vi "Tetra_BOUNCE_Payload.vi"(8 "error in":errorcluster, 10 "Input Constants":string[](array[string]), 11 "Parameters":string[](array[string])=["room", "18.75", "1", "0", "1", "15.5", "31.5"]) -> (0 "error out":errorcluster={"status"=FALSE, "code"=1073676294, "source"="VISA Read in Tetra Loop Serial.vi:4650001->Tetra_Read Imon.vi->Tetra_TX_Payload.vi"}, 2 "Payload Results":string[](array[string])=["0.000", "0.000", "0.000", "0.000", "0.000", "0.000", "0.000", "0.000", "-32.000", "1.000", "18.390", "0.998", "1.810", "3.312", "0.996", "1.198", "5.011", "3.316", "2.513", "2.513", "3.600", "5.496", "2.776", "2.768", "2.280", "1.360", "0.187", "0.089", "0.321", "0.340", "1.483", "0.530", "0.827", "7.000", "P0003", "trace file path"])   [LabVIEW 2018]
uses:
  778a857b-ea1c-4c41-85f0-8bde546241f8.vi
  e7e3a4d5-9ed6-4285-8f90-f7af1205463a.vi
  Initialize References/Station References Global.vi
  Initialize References/Sequence Globals.vi
  Tetra_Globals.vi
  Infrastructure/Test Parameter Globals_1.0.0.vi
  Infrastructure/Test Result File Name Global.vi
panel:
  in  "Controls":T1={"ReadADC"=TRUE, "StartTest"=TRUE, "ResetRFSM"=TRUE, "FtServer"=TRUE, "CalVCO(t)"=TRUE, "Ping(t)"=TRUE, "CmdWindowHide(T)"=FALSE, "OpenNewFt(T)"=TRUE, "UseCmdFile(T)"=FALSE, "#of Retries"=5}
  out "message":string="Scan Failed! Try to run vco cal, then press OK\nScan Failed! In Field Test ; Try to Terminate Scan, Then Prep for new scan"
  out "Pass?(T)":bool
  out "Current Iteration":i32=1
  out "PASS/FAIL":string
  out "DataToResultFile":string[][](array[string])
  out "no_fault":bool
  out "FH_NOT(T)":bool
  in  "ess_error":errorcluster
  out "STOP(T)":bool
  in  "Tab Control":enum32{"Page 1", "Page 2", "Page 3", "Page 4"}(tab)
  out "#OFAVGs":i32
  out "Temp Soak(min)":dbl
  in  "Standalone(T)":bool
  out "V_SUPPLY(t)":bool
  out "TEMP(t)":bool
  out "GET_TRACE":bool
  out "TEMP":dbl
  out "V_SUPPLY":dbl=18.75
  in  "CheckDataRetry(t)":bool
  out "ps_meas(i)(w)":dbl[](array[numeric])
  out "Ampl_Graph":dbl[][](graph)
  out "Freq_Graph":dbl[](graph)
  out "comport":refnum<visa-resource-name>
  out "CalFileA":path
  out "relative seconds":dbl=73640.4138221 format="%_19f"
  out "iq_file_str":string
  out "TraceFilePath":path
  out "Run_Clk_Test(t)":bool
  out "ClkTestPASS?(t)":bool
  out "PyScript(path)":path=path "C:/RageATE/Automated Tests/Tetra WAM/Utilities/VerifySiTime.py"
  out "WamGood(path)":path=path "C:/RageATE/Automated Tests/Tetra WAM/Utilities/ext_wamGood.txt"
  out "CLK_P/F(str)":string
  out "GuiPath":path
  out "FtPath":path
  # "Globals (last value change)"
  # "Vmon & Imon"
  # "Temp Sensors"
types:
  T1 = cluster{"ReadADC":bool, "StartTest":bool, "ResetRFSM":bool, "FtServer":bool, "CalVCO(t)":bool, "Ping(t)":bool, "CmdWindowHide(T)":bool, "OpenNewFt(T)":bool, "UseCmdFile(T)":bool, "#of Retries":i32}
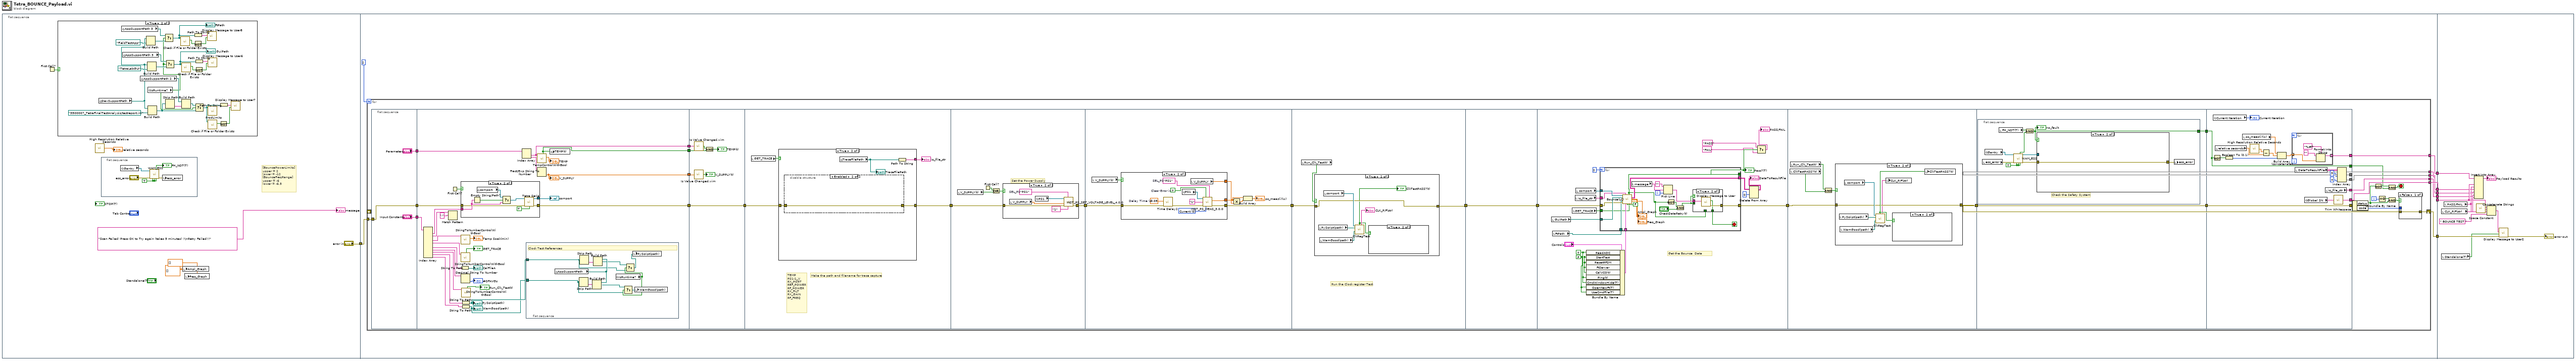
[diagram p0: block diagram]
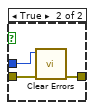
[diagram p3: hidden frame]
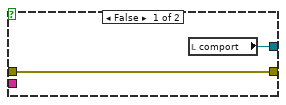
[diagram p4: hidden frame]
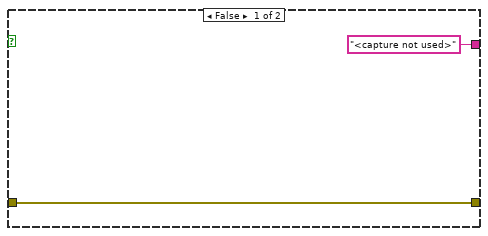
[diagram p5: hidden frame]
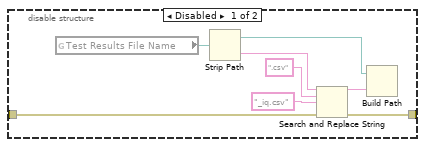
[diagram p6: hidden frame]
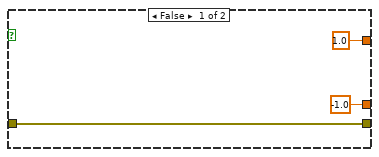
[diagram p8: hidden frame]
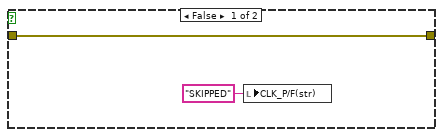
[diagram p9: hidden frame]
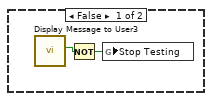
[diagram p10: hidden frame]
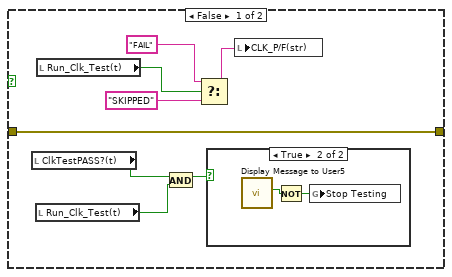
[diagram p12: hidden frame]
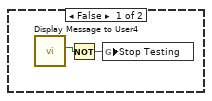
[diagram p14: hidden frame]
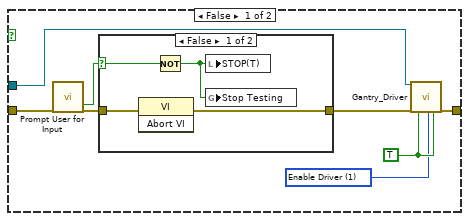
[diagram p15: hidden frame]
diagram:
  n1 = flat-sequence {
    tunnel: ["error in"] -> w5
    tunnel: [w51] -> w7
    tunnel: [w50] -> w6
    tunnel: w5 -> [w49]
    tunnel: [w47] -> w4
    tunnel: [w46] -> w3
    tunnel: [w45] -> w2
    tunnel: [w44] -> w1
    tunnel: w1 -> [w332]
    tunnel: w2 -> [w333]
    tunnel: w3 -> [w334]
    tunnel: w4 -> [w336]
    tunnel: w6 -> [w335]
    tunnel: w7 -> [w337]
    frame #0 {
      # "[BouncePowerLimits]\nupper = 2\nlower = -12\n[BounceFreqRange]\nupper = -6\nlower = -6.5"
      n2 = First Call?() -> (First Call?: T/F=w11:bool)
      n3 = case shown="True" w11 {
        frame False {
        }
        frame True {
          n4 = global read "Sequence Globals.vi" "DevSupportPath"() -> (w15:path)
          n5 = global read "Sequence Globals.vi" "AppSupportPath 3"() -> (w16:path)
          n6 = global read "Sequence Globals.vi" "AppSupportPath 3"() -> (w35:path)
          n7 = global read "Sequence Globals.vi" "AppSupportPath 2"() -> (w37:path)
          n8 = Build Path(base path=w15, name or relative path=path "FieldTestApp" ("*.ini file")) -> (appended path=w17:path)
          n9 = Build Path(base path=w15, name or relative path=path "TetraLabGUI" ("*.ini file")) -> (appended path=w32:path)
          n10 = global read "Sequence Globals.vi" "IsRuntime?"() -> (w14:bool)
          n11 = Build Path(base path=w15, name or relative path=path "3500007_TetraFinalTestAnalysis/testreport.ini" ("*.ini file")) -> (appended path=w34:path)
          n12 = Select(t=w16, s=w14, f=w17) -> (s? t:f=w19:path)
          "FtPath" <- w19
          n13 = Select(t=w35, s=w14, f=w32) -> (s? t:f=w30:path)
          "GuiPath" <- w30
          n14 = Strip Path(path=w34) -> (name=w38:string)  [unwired: 1 out]
          n15 = call <vilib>:"Check if File or Folder Exists.vi"("path"=w19) -> ("file or folder exists?"=w21:bool)  [unwired: 8 in, 2 out]
          n16 = call <vilib>:"Check if File or Folder Exists.vi"("path"=w30) -> ("file or folder exists?"=w24:bool)  [unwired: 8 in, 2 out]
          n17 = Build Path(base path=w37, name or relative path=w38) -> (appended path=w36:path)
          n18 = Path To String(path=w19) -> (string=w20:string)
          n19 = Not(x=w21) -> (.not. x?=w22:bool)
          n20 = Path To String(path=w30) -> (string=w29:string)
          n21 = Not(x=w24) -> (.not. x?=w23:bool)
          n22 = Select(t=w36, s=w14, f=w34) -> (s? t:f=w27:path)
          n23 = call "Display Message to User8"("Enable"=w22, "Message"=w20) -> ()  [unwired: 8 in, 2 out]
          n24 = call "Display Message to User6"("Enable"=w23, "Message"=w29) -> ()  [unwired: 8 in, 2 out]
          n25 = call "ProdLimits.vi"("*.ini file"=w27) -> ()  [unwired: 9 in, 2 out]
          n26 = call <vilib>:"Check if File or Folder Exists.vi"("path"=w27) -> ("file or folder exists?"=w26:bool)  [unwired: 8 in, 2 out]
          n27 = Path To String(path=w27) -> (string=w28:string)
          n28 = Not(x=w26) -> (.not. x?=w25:bool)
          n29 = call "Display Message to User7"("Enable"=w25, "Message"=w28) -> ()  [unwired: 8 in, 2 out]
        }
      }
      n30 = call <vilib>:"High Resolution Relative Seconds.vi"() -> ("relative seconds"=→"relative seconds":dbl)
      n31 = flat-sequence {
        frame #0 {
          w41 = TRUE ("Test Running (T)")
          n32 = global read "Station References Global.vi" "Gantry"() -> (w42:refnum<visa-resource-name>)
          n33 = call "WAM_ESS.vi"("VISA resource name"=w42, "error in (no error)"="ess_error", "Open Serial"=w41, "Test Running (T)"=w41, "Close Serial"=w41) -> ("FH_NOT(T)"=→"FH_NOT(T)":bool, "error out"=w39:errorcluster)  [unwired: 7 in, 2 out]
          n34 = local write "ess_error"(w39) -> ()
        }
      }
      n35 = local write "Ampl_Graph"(dbl[][] [] ("Ampl_Graph")) -> ()
      n36 = local write "Freq_Graph"(dbl[] [] ("Freq_Graph")) -> ()
      "message" <- "Scan Failed! Press OK to Try again (takes 5 minutes) !!\nRetry Failed!!!" ("multi-line string")
    }
    frame #1 {
      n37 = for {
        N: 2 -> [_]
        tunnel: [w75] -> w51
        tunnel: [w74] -> w50
        tunnel: w49 -> [w73]
        shift-right: [w68] -> w47
        shift-left: _ -> [_]
        tunnel: [w61] -> w46
        tunnel: [w60] -> w45
        tunnel: [w59] -> w44
        i -> [w65]
        stop <- w71 stop-if-true
        n38 = flat-sequence {
          tunnel: [w89] -> w84
          tunnel: ["Parameters"] -> w83
          tunnel: ["Input Constants"] -> w82
          tunnel: w73 -> [w89]
          tunnel: w84 -> [w100]
          tunnel: [w99] -> w81
          tunnel: w83 -> [w114]
          tunnel: w82 -> [w113]
          tunnel: [w112] -> w80
          tunnel: [w109] -> w79
          tunnel: [w104] -> w78
          tunnel: [w146] -> w77
          tunnel: w78 -> [w140]
          tunnel: w79 -> [w142]
          tunnel: w80 -> [w144]
          tunnel: w81 -> [w146]
          tunnel: [w149] -> w72
          tunnel: w77 -> [w148]
          tunnel: [w170] -> w76
          tunnel: w72 -> [w168]
          tunnel: [w184] -> w55
          tunnel: w76 -> [w183]
          tunnel: w55 -> [w201]
          tunnel: [w200] -> w54
          tunnel: w54 -> [w212]
          tunnel: [w212] -> w58
          tunnel: [w229] -> w53
          tunnel: w58 -> [w231]
          tunnel: w53 -> [w260]
          tunnel: [w261] -> w52
          tunnel: w52 -> [w280]
          tunnel: [w281] -> w62
          tunnel: [w280] -> w56
          tunnel: [w315] -> w67
          tunnel: [w320] -> w75
          tunnel: [w317] -> w74
          tunnel: w62 -> [w305]
          tunnel: [w310] -> w61
          tunnel: [w308] -> w60
          tunnel: [w307] -> w59
          tunnel: [w305] -> w57
          tunnel: w56 -> [w315]
          frame #0 {
          }
          frame #1 {
            n39 = Index Array(array=w113) -> (element #1=w102:string, element #2=w105:string, element #4=w119:string, element #5=w98:string, element #7=w116:string, element #8=w111:string, element #9=w97:string, element #10=w95:string, element #11=w94:string)  [unwired: 11 in, 2 out]
            n40 = Match Pattern(string=w105, regular expression=";") -> ()  [unwired: 1 in, 4 out]
            n41 = First Call?() -> (First Call?: T/F=w101:bool)
            n42 = String To Path(string=w116) -> (path=→"CalFileA":path)
            n43 = case shown="True" w101 {
              tunnel: [w131 w135] -> w103
              tunnel: w102 -> [_ w137]
              tunnel: w100 -> [w130 w134]
              tunnel: [w130 w133] -> w99
              frame False {
                n44 = local read "comport"() -> (w131:refnum<visa-resource-name>)
              }
              frame True {
                n45 = Empty String/Path?(string/path=w137) -> (empty?=w139:bool)
                n46 = global read "Tetra_Globals.vi" "comport"() -> (w138:refnum<visa-resource-name>)
                n47 = Select(t=w138, s=w139, f=w137) -> (s? t:f=w136:refnum<visa-resource-name>)
                n48 = call "Tetra Serial.vi"("COMPORT"=w136, "error in (no error)"=w134, "Open Ser(t)"=TRUE) -> ("comport"=w135:refnum<visa-resource-name>, "error out"=w133:errorcluster)  [unwired: 8 in, 3 out]
              }
            }
            "comport" <- w103
            n49 = call "StringToNumberControlWithBool.vi"("String In"=w119) -> ("Number Out"=→"Temp Soak(min)":dbl)  [unwired: 7 in, 1 out]
            n50 = call "StringToNumberControlWithBool.vi"("String In"=w98) -> ("NOT = 0"=→"GET_TRACE":bool)  [unwired: 7 in, 1 out]
            n51 = Decimal String To Number(string=w111) -> (number=→"#OFAVGs":i32)  [unwired: 2 in, 1 out]
            n52 = String To Path(string=w95) -> (path=w93:path)
            "PyScript(path)" <- w93
            n53 = String To Path(string=w94) -> (path=w92:path)
            "WamGood(path)" <- w92
            n54 = call "StringToNumberControlWithBool.vi"("String In"=w97) -> ("NOT = 0"=→"Run_Clk_Test(t)":bool)  [unwired: 7 in, 1 out]
            n55 = Index Array(array=w114) -> (element #1=w109:string, element #2=w118:string)  [unwired: 2 in]
            n56 = flat-sequence {
              tunnel: w93 -> [w121]
              tunnel: w92 -> [w120]
              frame #0 {
                # "Clock Test References"
                n57 = global read "Sequence Globals.vi" "AppSupportPath"() -> (w127:path)
                n58 = Strip Path(path=w120) -> (name=w128:string)  [unwired: 1 out]
                n59 = Strip Path(path=w121) -> (name=w129:string)  [unwired: 1 out]
                n60 = Build Path(base path=w127, name or relative path=w128) -> (appended path=w125:path)
                n61 = Build Path(base path=w127, name or relative path=w129) -> (appended path=w126:path)
                n62 = global read "Sequence Globals.vi" "IsRuntime?"() -> (w124:bool)
                n63 = Select(t=w125, s=w124, f=w120) -> (s? t:f=w122:path)
                n64 = Select(t=w126, s=w124, f=w121) -> (s? t:f=w123:path)
                n65 = local write "PyScript(path)"(w123) -> ()
                n66 = local write "WamGood(path)"(w122) -> ()
              }
            }
            n67 = call "TempControlWithBool.vi"("INPUT"=w109) -> ("out"=→"TEMP":dbl, "Valid(t)"=w104:bool)  [unwired: 6 in, 1 out]
            n68 = Fract/Exp String To Number(string=w118) -> (number=w112:dbl)  [unwired: 3 in, 1 out]
            "V_SUPPLY" <- w112
            n69 = global write "Tetra_Globals.vi" "TEMP(t)"(w104) -> ()
          }
          frame #2 {
            n70 = call "Is Value Changed.vim"("value"=w142) -> ("changed or first call?"=w143:bool)
            n71 = call "Is Value Changed.vim"("value"=w144) -> ("changed or first call?"=→"V_SUPPLY(t)":bool)
            n72 = And(x=w143, y=w140) -> (x .and. y?=→"TEMP(t)":bool)
          }
          frame #3 {
            # "TEMP\nPS1-1_V\nRX_PORT\nREF_POWER\nRF_POWER\nRX_FILT\nRX_GAIN\nRF_FREQ"
            # "Make the path and filename for trace capture"
            n73 = local read "GET_TRACE"() -> (w150:bool)
            n74 = case shown="True" w150 {
              tunnel: [w152 w155] -> w149
              tunnel: w148 -> [w152 w156]
              tunnel: ["<capture not used>" w154] -> w147
              frame False {
              }
              frame True {
                n75 = disable-structure shown="Enabled" {
                  disable-tunnel: w156 -> [w158 w165]
                  disable-tunnel: [w157 w165] -> w155
                  frame Disabled {
                    n76 = global read "Test Result File Name Global.vi" "Test Results File Name"() -> (w161:path)
                    n77 = Strip Path(path=w161) -> (stripped path=w162:path, name=w164:string)
                    n78 = Search and Replace String(input string=w164, search string=".csv", replace string="_iq.csv" ("name or relative path"), error in=w158) -> (result string=w163:string, error out=w157:errorcluster)  [unwired: 4 in, 2 out]
                    n79 = Build Path(base path=w162, name or relative path=w163) -> ()  [unwired: 1 out]
                  }
                  frame Enabled {
                  }
                }
                n80 = global read "Tetra_Globals.vi" "TraceFilePath"() -> (w153:path)
                "TraceFilePath" <- w153
                n81 = Path To String(path=w153) -> (string=w154:string)
              }
            }
            "iq_file_str" <- w147
          }
          frame #4 {
            # "Set the Power Supply"
            n82 = local read "V_SUPPLY(t)"() -> (w169:bool)
            n83 = First Call?() -> (First Call?: T/F=w167:bool)
            n84 = Or(x=w167, y=w169) -> (x .or. y?=w166:bool)
            n85 = case shown="True" w166 {
              tunnel: [w171 w173] -> w170
              tunnel: w168 -> [w171 w172]
              frame False {
              }
              frame True {
                w176 = "PS1"  # SEL_PS
                n86 = local read "V_SUPPLY"() -> (w175:dbl)
                n87 = global read "Station References Global.vi" "PS1"() -> (w177:refnum<visa-resource-name>)
                n88 = call "INST_PS_SET_VOLTAGE_LEVEL_4.0.0.vi"("Instrument Select (Output 1)"="1", "SEL_PS"=w176, "error in (no error)"=w172, "Voltage (0.0)"=w175, "VISA session"=w177) -> ("error out"=w173:errorcluster)  [unwired: 5 in, 1 out]
              }
            }
          }
          frame #5 {
            n89 = local read "V_SUPPLY(t)"() -> (w178:bool)
            n90 = case shown="True" w178 {
              tunnel: [-1.0 w189] -> w180
              tunnel: [w187 w190] -> w184
              tunnel: w183 -> [w187 w191]
              tunnel: [1.0 ("V_SUPPLY") w188] -> w182
              frame False {
              }
              frame True {
                w192 = TRUE  # Clear Error in
                w193 = 0.05  # Delay Time (s)
                w197 = 0 items=["Current", "Voltage"] ("Measurement Type (1: Voltage)")
                w198 = "PS1"  # SEL_PS
                n91 = call "Time Delay2"("error in (no error)"=w191, "Delay Time (s)"=w193) -> ("error out"=w194:errorcluster)  [unwired: 9 in]
                n92 = global read "Station References Global.vi" "PS1"() -> (w195:refnum<visa-resource-name>)
                n93 = local read "V_SUPPLY"() -> (w188:dbl)
                n94 = call "INST_PS_MEAS_3.0.0.vi"("VISA session"=w195, "Clear Error in"=w192, "SEL_PS"=w198, "Channel Name (1)"="1", "error in (no error)"=w194, "Measurement Type (1: Voltage)"=w197) -> ("Measurement"=w189:dbl, "error out"=w190:errorcluster)  [unwired: 6 in, 2 out]
              }
            }
            n95 = Multiply(x=w180, y=w182) -> (x*y=w181:dbl)
            n96 = Build Array(w180, w181) -> (→"ps_meas(i)(w)":dbl[])
          }
          frame #6 {
            # "Run the Clock register Test"
            n97 = local read "Run_Clk_Test(t)"() -> (w199:bool)
            n98 = case shown="True" w199 {
              tunnel: [w203 w206] -> w200
              tunnel: w201 -> [w203 w206]
              frame False {
                n99 = local write "CLK_P/F(str)"("SKIPPED" ("CLK_P/F(str)")) -> ()
              }
              frame True {
                n100 = local read "PyScript(path)"() -> (w207:path)
                n101 = local read "WamGood(path)"() -> (w208:path)
                n102 = local read "comport"() -> (w209:refnum<visa-resource-name>)
                n103 = call "ClkRegTest.vi"("COMPORT"=w209, "PyScript(path)"=w207, "WamGood(path)"=w208) -> ("P/F(bool)"=w204:bool, "P/F(str)"=→"CLK_P/F(str)":string)  [unwired: 9 in, 2 out]
                "ClkTestPASS?(t)" <- w204
                n104 = case shown="True" w204 {
                  frame False {
                    n105 = call "Display Message to User3"() -> ("OK"=w211:bool)  [unwired: 10 in, 1 out]
                    n106 = Not(x=w211) -> (.not. x?=w210:bool)
                    n107 = global write "Sequence Globals.vi" "Stop Testing"(w210) -> ()
                  }
                  frame True {
                  }
                }
              }
            }
          }
          frame #7 {
          }
          frame #8 {
            w216 = FALSE ("StartTest")
            w217 = TRUE ("ReadADC")
            # "Get the Bounce  Data"
            n108 = local read "GuiPath"() -> (w226:path)
            n109 = local read "FtPath"() -> (w224:path)
            n110 = local read "GET_TRACE"() -> (w227:bool)
            n111 = local read "iq_file_str"() -> (w228:string)
            n112 = local read "comport"() -> (w225:refnum<visa-resource-name>)
            n113 = Bundle By Name(cluster="Controls", "ReadADC"=w217, "StartTest"=w216, "ResetRFSM"=w216, "FtServer"=w216, "CalVCO(t)"=w216, "Ping(t)"=w217, "CmdWindowHide(T)"=w217, "OpenNewFt(T)"=w216, "UseCmdFile(T)"=w216) -> (w222:T1)
            n114 = for {
              N: 2 ("#OFAVGs") -> [_]
              tunnel: [w252] -> w229
              tunnel: w231 -> [w243]
              tunnel: w228 -> [w236]
              tunnel: w227 -> [w235]
              tunnel: [w232] -> w220
              tunnel: w226 -> [w244]
              tunnel: w225 -> [w245]
              tunnel: w224 -> [w242]
              tunnel: [w241] -> w215
              tunnel: w222 -> [w239]
              i -> [w251]
              stop <- w233 stop-if-true
              n115 = call "Bounce(LC).vi"("COMPORT"=w245, "i/q_file"=w236, "Gui(path)"=w244, "Ft directory"=w242, "error in (no error)"=w243, "Controls"=w239, "Standalone vi(t)"=FALSE, "Write i/q data file"=w235) -> ("P/F Bounce"=w232:bool, "Data_Out"=w241:string[][], "Ampl_Graph"=→"Ampl_Graph":dbl[][], "Freq_Graph"=→"Freq_Graph":dbl[])  [unwired: 2 in, 2 out]
              n116 = local read "message"() -> (w250:string)
              n117 = Pick Line(string ("")="", multi-line string=w250, line index=w251) -> (output string=w248:string)
              n118 = Not(x=w232) -> (.not. x?=w247:bool)
              n119 = And(x=w247, y="CheckDataRetry(t)") -> (x .and. y?=w234:bool)
              n120 = case shown="True" w234 {
                tunnel: [_ w256] -> w252
                tunnel: w248 -> [_ w255]
                tunnel: w234 -> [_ _]
                tunnel: [w253 w254] -> w233
                tunnel: w232 -> [w253 _]
                frame False {
                }
                frame True {
                  n121 = call "Display Message to User"("Message"=w255) -> ("error out"=w256:errorcluster, "Cancel"=w254:bool)  [unwired: 9 in]
                }
              }
            }
            "Pass?(T)" <- w220
            n122 = Delete From Array(array=w215, index (row)=0) -> (array with subset deleted=→"DataToResultFile":string[][])  [unwired: 2 in, 1 out]
            n123 = Select(t="PASS", s=w220, f="FAIL") -> (s? t:f=→"PASS/FAIL":string)
          }
          frame #9 {
            n124 = local read "ClkTestPASS?(t)"() -> (w257:bool)
            n125 = local read "Run_Clk_Test(t)"() -> (w259:bool)
            n126 = And(x=w259, y=w257) -> (x .and. y?=w258:bool)
            n127 = case shown="True" w258 {
              tunnel: [w269 w273] -> w261
              tunnel: w260 -> [w269 w273]
              frame False {
                n128 = local read "ClkTestPASS?(t)"() -> (w264:bool)
                n129 = local read "Run_Clk_Test(t)"() -> (w262:bool)
                n130 = local read "Run_Clk_Test(t)"() -> (w265:bool)
                n131 = And(x=w264, y=w262) -> (x .and. y?=w263:bool)
                n132 = Select(t="FAIL" ("CLK_P/F(str)"), s=w265, f="SKIPPED" ("CLK_P/F(str)")) -> (s? t:f=w268:string)
                n133 = case shown="True" w263 {
                  frame False {
                  }
                  frame True {
                    n134 = call "Display Message to User5"() -> ("OK"=w271:bool)  [unwired: 10 in, 1 out]
                    n135 = Not(x=w271) -> (.not. x?=w270:bool)
                    n136 = global write "Sequence Globals.vi" "Stop Testing"(w270) -> ()
                  }
                }
                n137 = local write "CLK_P/F(str)"(w268) -> ()
              }
              frame True {
                n138 = local read "PyScript(path)"() -> (w275:path)
                n139 = local read "WamGood(path)"() -> (w276:path)
                n140 = local read "comport"() -> (w277:refnum<visa-resource-name>)
                n141 = call "ClkRegTest.vi"("COMPORT"=w277, "PyScript(path)"=w275, "WamGood(path)"=w276) -> ("P/F(bool)"=w274:bool, "P/F(str)"=w272:string)  [unwired: 9 in, 2 out]
                n142 = local write "CLK_P/F(str)"(w272) -> ()
                n143 = case shown="True" w274 {
                  frame False {
                    n144 = call "Display Message to User4"() -> ("OK"=w279:bool)  [unwired: 10 in, 1 out]
                    n145 = Not(x=w279) -> (.not. x?=w278:bool)
                    n146 = global write "Sequence Globals.vi" "Stop Testing"(w278) -> ()
                  }
                  frame True {
                  }
                }
                n147 = local write "ClkTestPASS?(t)"(w274) -> ()
              }
            }
          }
          frame #10 {
            n148 = flat-sequence {
              tunnel: [w283] -> w281
              frame #0 {
                w284 = TRUE ("Close Serial")
                # "Check the Safety System"
                n149 = local read "ess_error"() -> (w289:errorcluster)
                n150 = global read "Station References Global.vi" "Gantry"() -> (w287:refnum<visa-resource-name>)
                n151 = local read "FH_NOT(T)"() -> (w286:bool)
                n152 = call "WAM_ESS.vi"("VISA resource name"=w287, "error in (no error)"=w289, "Open Serial"=w284, "Test Running (T)"=w284, "Close Serial"=w284) -> ("FH_NOT(T)"=w285:bool, "VISA resource name out"=w288:refnum<visa-resource-name>, "error out"=w290:errorcluster)  [unwired: 7 in, 1 out]
                n153 = And(x=w286, y=w285) -> (x .and. y?=w283:bool)
                "no_fault" <- w283
                n154 = case shown="True" w283 {
                  tunnel: w288 -> [w298 _]
                  tunnel: w290 -> [w297 w304]
                  tunnel: [w296 w304] -> w282
                  frame False {
                    w294 = u16 1 items=["Disable Driver", "Enable Driver", "Read Driver Status"] ("Driver-Func")
                    w295 = TRUE ("Close Serial")
                    n155 = call "Prompt User for Input"("error in (no error)"=w297) -> ("OK"=w293:bool, "error out"=w292:errorcluster)  [unwired: 17 in]
                    n156 = case shown="False" w293 {
                      selector: w293 -> [w300 _]
                      tunnel: w292 -> [w302 w303]
                      tunnel: [w301 w303] -> w291
                      frame False {
                        n157 = invoke class="VI" method="Abort VI"(error in=w302) -> (error out=w301:errorcluster)  [unwired: 2 in, 2 out]
                        n158 = Not(x=w300) -> (.not. x?=w299:bool)
                        n159 = local write "STOP(T)"(w299) -> ()
                        n160 = global write "Sequence Globals.vi" "Stop Testing"(w299) -> ()
                      }
                      frame True {
                      }
                    }
                    n161 = call "Gantry_Driver.vi"("VISA resource name"=w298, "error in (no error)"=w291, "Open Serial"=w295, "Driver-Func"=w294, "Close Serial"=w295) -> ("error out"=w296:errorcluster)  [unwired: 11 in, 3 out]
                  }
                  frame True {
                  }
                }
                n162 = local write "ess_error"(w282) -> ()
              }
            }
          }
          frame #11 {
            n163 = Not(x=w305) -> (.not. x?=w306:bool)
            n164 = global read "Sequence Globals.vi" "Current Iteration"() -> (→"Current Iteration":i32)
            n165 = local read "relative seconds"() -> (w322:dbl)
            n166 = Boolean To (0,1)(Boolean=w306) -> (0, 1=w316:i16)
            n167 = local read "ps_meas(i)(w)"() -> (w314:dbl[])
            n168 = call <vilib>:"High Resolution Relative Seconds.vi"() -> ("relative seconds"=w323:dbl)
            n169 = Subtract(x=w323, y=w322) -> (x-y=w321:dbl)
            n170 = Build Array (concatenate)(w314, w321, w316) -> (w318:dbl[])
            n171 = for {
              tunnel: w318 -> [w325] mode=indexing
              tunnel: [w324] -> w317 mode=indexing
              n172 = Format Into String(format string="%#f", initial string="", w325) -> (resulting string=w324:string)  [unwired: 1 in, 1 out]
            }
            n173 = local read "DataToResultFile"() -> (w312:string[][])
            n174 = global read "Test Parameter Globals_1.0.0.vi" "Global SN"() -> (w319:string)
            n175 = local read "iq_file_str"() -> (w307:string)
            n176 = call <vilib>:"Trim Whitespace.vi"("string"=w319) -> ("trimmed string"=w320:string)  [unwired: 1 in]
            n177 = Index Array(array=w312, index (col) #1=3 ("disabled index (col)"), index (col) #2=4 ("index (col)")) -> (element #1=w310:string[], element #2=w308:string[])  [unwired: 2 in]
          }
        }
        n178 = Unbundle By Name(w67) -> ("status"=w66:bool, "code"=w69:i32)
        n179 = Not(x=w66) -> (.not. x?=w70:bool)
        n180 = Equal To 0?(x=w65) -> (x = 0?=w63:bool)
        n181 = And(x=w70, y=w57) -> (x .and. y?=w71:bool)
        n182 = And(x=w63, y=w66) -> (x .and. y?=w64:bool)
        n183 = case shown="False" w64 {
          tunnel: w69 -> [_ w88]
          tunnel: [w85 w87] -> w68
          tunnel: w67 -> [w85 w86]
          frame False {
          }
          frame True {
            n184 = call <vilib>:"Clear Errors.vi"("error in (no error)"=w86, "specific error code to clear (0: all)"=w88) -> ("error out"=w87:errorcluster)  [unwired: 4 in, 1 out]
          }
        }
      }
    }
    frame #2 {
      n185 = local read "CLK_P/F(str)"() -> (w328:string)
      n186 = local read "Standalone(T)"() -> (w329:bool)
      n187 = local read "PASS/FAIL"() -> (w330:string)
      n188 = Insert Into Array(array=w335, new element #1=w337, new element #2=w330, new element #3=w334, new element #4=w333, new element #5=w332, new element #6=w328) -> (→"Payload Results":string[])  [unwired: 1 in]
      n189 = call <vilib>:"Space Constant.vi"() -> ("String"=w339:string)
      n190 = Concatenate Strings(w337, w339, w330, " BOUNCE TEST " ("string")) -> (w340:string)
      n191 = call "Display Message to User2"("error in (no error)"=w336, "Enable"=w329, "Message"=w340) -> ("error out"=→"error out":errorcluster)  [unwired: 7 in, 1 out]
    }
  }
